vi "validate.vi"(8 "error in":errorcluster, 11 "configuration in":refnum<class "TBM module configuration.lvclass">) -> (0 "error out":errorcluster, 3 "configuration out":refnum<class "TBM module configuration.lvclass">)   [LabVIEW 2013, in "TBM module configuration.lvclass"]
doc: "Provides an interface for performing validation on a given configuration. Any children should define the behavior of this function to ensure that the configuration in memory can be used by the runtime class."
uses:
  TBM module configuration.lvclass
  root configuration/TBM configuration.lvclass
  <vilib>/NI/Tag Bus/tag/tag descriptor.lvclass/tag descriptor.ctl
  channel/TBM channel.lvclass/TBM channel.ctl
  <vilib>/NI/Tag Bus/tag/read tag name.vi
  <vilib>/NI/Tag Bus/tag/read data type.vi
  channel/Read channel classification.vi
  channel/TBM channel.lvclass
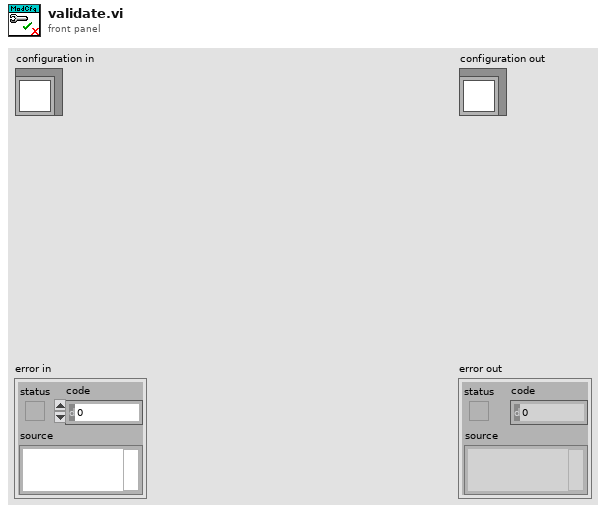
[diagram p1: front panel]
types:
  T1 = typedef "TBM channel.lvclass/channel classification.ctl" = enum16{"input data", "output data", "processing parameter", "processing result"}
  T2 = typedef "tag bus.lvlib/tag descriptor.lvclass/Data Type.ctl" = enum16{"Double", "Single", "I64", "I32", "I16", "I8", "U64", "U32", "U16", "U8", "Boolean", "String", "Array of Double", "Array of Single", "Array of I64", "Array of I32", "Array of I16", "Array of I8", "Array of U64", "Array of U32", "Array of U16", "Array of U8", "Array of Boolean", "Array of String"}
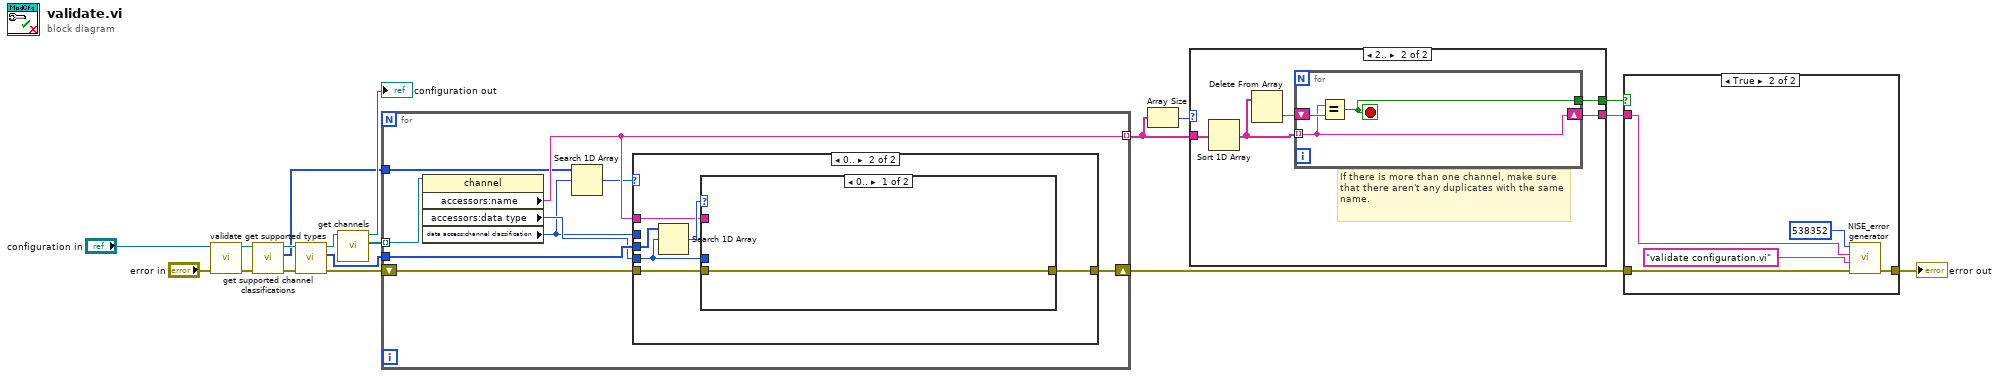
[diagram p0: block diagram]
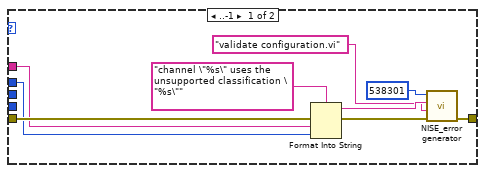
[diagram p4: hidden frame]
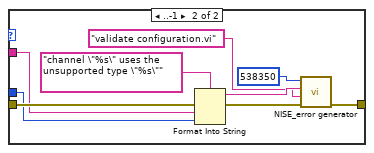
[diagram p5: hidden frame]
diagram:
  n1 = call-parent "validate.vi"("error in"="error in", "configuration in"="configuration in") -> ("error out"=w16:errorcluster, "configuration out"=w3:refnum<class "TBM module configuration.lvclass">)  [unwired: 8 in]
  n2 = call-dynamic "get supported channel classifications.vi"("error in"=w16, "module configuration in"=w3) -> ("error out"=w4:errorcluster, "supported types"=w1:T1[], "module configuration out"=w2:refnum<class "TBM module configuration.lvclass">)  [unwired: 7 in]
  n3 = call-dynamic "get supported types.vi"("error in"=w4, "module configuration in"=w2) -> ("error out"=w12:errorcluster, "supported types"=w13:T2[], "module configuration out"=w15:refnum<class "TBM module configuration.lvclass">)  [unwired: 7 in]
  n4 = call-dynamic "get channels.vi"("module configuration in"=w15) -> ("channels"=w14:refnum<class "TBM channel.lvclass">[], "module configuration out"=→"configuration out":refnum<class "TBM module configuration.lvclass">)  [unwired: 9 in]
  n5 = for {
    tunnel: w14 -> [w27] mode=indexing
    tunnel: w13 -> [w26]
    shift-right: [w24] -> w9
    shift-left: w12 -> [w25]
    tunnel: [w22] -> w6 mode=indexing
    tunnel: w1 -> [w21]
    n6 = property class="channel"(reference=w27) -> ("accessors:name"=w22:string, "accessors:data type"=w23:T2, "data access:channel classification"=w19:T1)  [unwired: 1 in, 2 out]
    n7 = Search 1D Array(1D array=w21, element=w19) -> (index of element=w20:i32)  [unwired: 1 in]
    n8 = case shown="0.." w20 {
      tunnel: w26 -> [_ w42]
      tunnel: w25 -> [w32 w40]
      tunnel: [w31 w39] -> w24
      tunnel: w23 -> [_ w38]
      tunnel: w22 -> [w28 w37]
      tunnel: w19 -> [w29 _]
      frame ..-1 {
        n9 = Format Into String(format string="channel \"%s\" uses the unsupported classification \"%s\"", error in=w32, w28, w29) -> (resulting string=w34:string, error out=w35:errorcluster)  [unwired: 1 in]
        n10 = call <vilib>:"NISE_error generator.vi"("error in"=w35, "source"="validate configuration.vi" ("format string"), "append error message"=w34, "error code (0)"=538301) -> ("error out"=w31:errorcluster)  [unwired: 5 in]
      }
      frame 0.. {
        n11 = Search 1D Array(1D array=w42, element=w38) -> (index of element=w41:i32)  [unwired: 1 in]
        n12 = case shown="0.." w41 {
          tunnel: w40 -> [w43 w47]
          tunnel: [w43 w46] -> w39
          tunnel: w38 -> [_ w45]
          tunnel: w37 -> [_ w44]
          frame 0.. {
          }
          frame ..-1 {
            n13 = Format Into String(format string="channel \"%s\" uses the unsupported type \"%s\"", error in=w47, w44, w45) -> (resulting string=w50:string, error out=w51:errorcluster)  [unwired: 1 in]
            n14 = call <vilib>:"NISE_error generator.vi"("error in"=w51, "source"="validate configuration.vi" ("format string"), "append error message"=w50, "error code (0)"=538350) -> ("error out"=w46:errorcluster)  [unwired: 5 in]
          }
        }
      }
    }
  }
  n15 = Array Size(array=w6) -> (size(s)=w5:i32)
  n16 = case shown="2.." w5 {
    tunnel: [_ w55] -> w8
    tunnel: [_ w54] -> w7
    tunnel: w6 -> [_ w53]
    frame ..1 {
    }
    frame 2.. {
      # "If there is more than one channel, make sure that there aren't any duplicates with the same name."
      n17 = Sort 1D Array(array=w53) -> (sorted array=w56:string[])
      n18 = Delete From Array(array=w56) -> (deleted portion=w57:string)  [unwired: 2 in, 1 out]
      n19 = for {
        shift-right: [w59] -> w54
        shift-left: w57 -> [w60]
        tunnel: w56 -> [w59] mode=indexing
        tunnel: [w58] -> w55
        stop <- w58 stop-if-true
        n20 = Equal?(x=w59, y=w60) -> (x = y?=w58:bool)
      }
    }
  }
  n21 = case shown="True" w8 {
    tunnel: w9 -> [w61 w65]
    tunnel: [w61 w66] -> w10
    tunnel: w7 -> [_ w64]
    frame False {
    }
    frame True {
      n22 = call <vilib>:"NISE_error generator.vi"("error in"=w65, "source"="validate configuration.vi" ("format string"), "append error message"=w64, "error code (0)"=538352) -> ("error out"=w66:errorcluster)  [unwired: 5 in]
    }
  }
  "error out" <- w10
